vi "WRAPPER_Playback.vi"() -> ()   [LabVIEW 2013]
panel:
  out "Array":cluster{path, "error constant":errorcluster}[](array[cluster])
  out "Currently Running":path
  out "size(s)":i32
  in  "Auto Folder Path":path=path "E:/Scrubbing/Auto"
  out "All VIs in Auto Dir":path[](array[path])
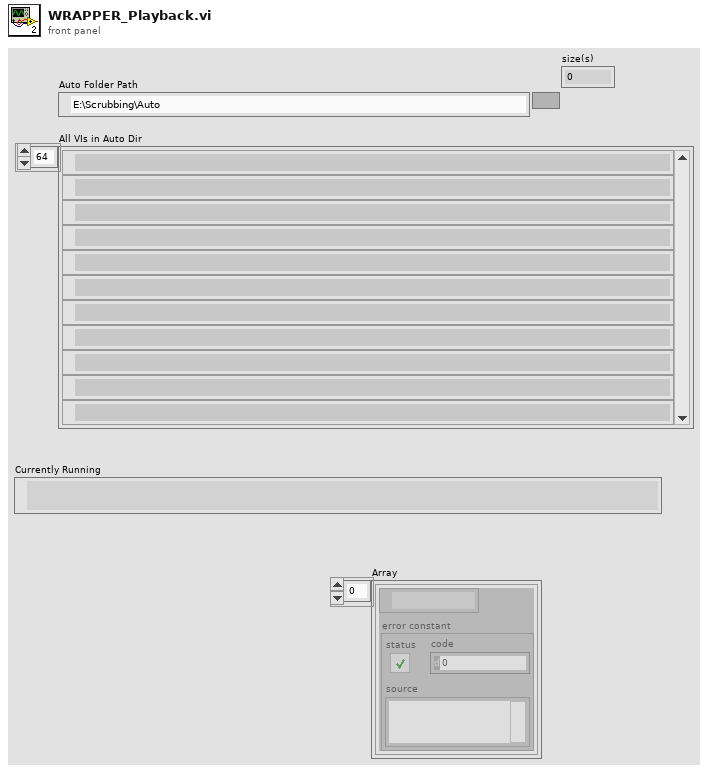
[diagram p1: front panel]
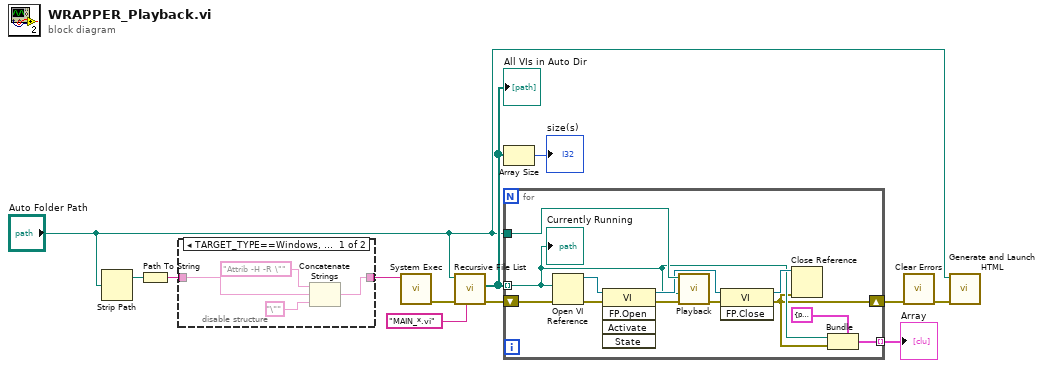
[diagram p0: block diagram]
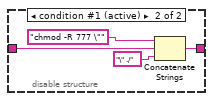
[diagram p2: hidden frame]
diagram:
  n1 = Strip Path(path="Auto Folder Path") -> (stripped path=w4:path)  [unwired: 1 out]
  n2 = Path To String(path=w4) -> (string=w3:string)
  n3 = disable-structure shown="TARGET_TYPE==Windows, Default" {
    disable-tunnel: w3 -> [w15 w19]
    disable-tunnel: [w13 w17] -> w2
    frame condition #0 {
      n4 = Concatenate Strings("Attrib -H -R \"" ("string"), w15, "\"" ("string")) -> (w13:string)
    }
    frame condition #1 (active) {
      n5 = Concatenate Strings("chmod -R 777 \"" ("string"), w19, "\" ./" ("string")) -> (w17:string)
    }
  }
  n6 = call <vilib>:"System Exec.vi"("command line"=w2) -> ("error out"=w1:errorcluster)  [unwired: 7 in, 3 out]
  n7 = call <vilib>:"Recursive File List.vi"("pattern"="MAIN_*.vi", "error in (no error)"=w1, "Folder Path"="Auto Folder Path") -> ("error out"=w8:errorcluster, "All Files in Dir"=w11:path[])  [unwired: 4 in, 3 out]
  "All VIs in Auto Dir" <- w11
  n8 = Array Size(array=w11) -> (size(s)=→"size(s)":i32)
  n9 = for {
    tunnel: "Auto Folder Path" -> [w32]
    tunnel: w11 -> [w24] mode=indexing
    tunnel: [w23] -> w9 mode=indexing
    shift-right: [w22] -> w7
    shift-left: w8 -> [w21]
    n10 = Open VI Reference(vi path=w24, error in (no error)=w21) -> (vi reference=w31:refnum<vi>, error out=w30:errorcluster)  [unwired: 4 in]
    n11 = invoke class="VI" method="FP.Open"(reference=w31, error in=w30) -> (reference out=w27:refnum<vi>, error out=w29:errorcluster)  [unwired: 3 in, 3 out]
    n12 = call "Playback.vi"("error in (no error)"=w29, "vi path"=w24, "Auto Folder Path"=w32) -> ("error out"=w28:errorcluster)  [unwired: 8 in]
    n13 = invoke class="VI" method="FP.Close"(reference=w27, error in=w28) -> (reference out=w26:refnum<vi>, error out=w22:errorcluster)  [unwired: 1 in, 1 out]
    n14 = Close Reference(reference=w26, error in (no error)=w22) -> ()  [unwired: 1 out]
    n15 = Bundle(cluster=cluster{path, "error constant":errorcluster} {path "", "error constant"={"status"=FALSE, "code"=0, "source"=""}}, w24, "error constant"=w22) -> (w23:cluster{path, "error constant":errorcluster})
    "Currently Running" <- w24
  }
  "Array" <- w9
  n16 = call <vilib>:"Clear Errors.vi"("error in (no error)"=w7) -> ("error out"=w6:errorcluster)  [unwired: 6 in]
  n17 = call "Generate and Launch HTML.vi"("error in"=w6, "Path"="Auto Folder Path") -> ()  [unwired: 9 in, 1 out]
